vi "2D array sum using for loop.vi"() -> ()   [LabVIEW 2010]
uses:
  <vilib>/Analysis/Matrix/Datatypes/RealMatrix.ctl
  <vilib>/Analysis/Matrix/NI_Matrix.lvlib
panel:
  out "Real Matrix":T1
  in  "Array2":T1
  in  "Array1":T1
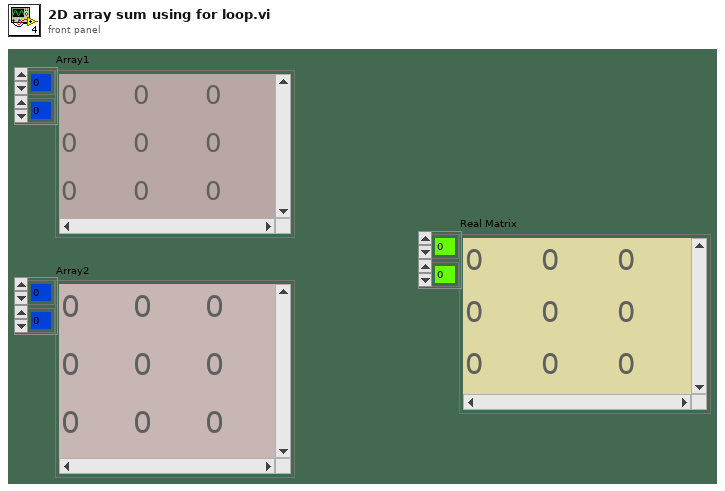
[diagram p1: front panel]
types:
  T1 = typedef "NI_Matrix.lvlib/RealMatrix.ctl" = dbl[][]
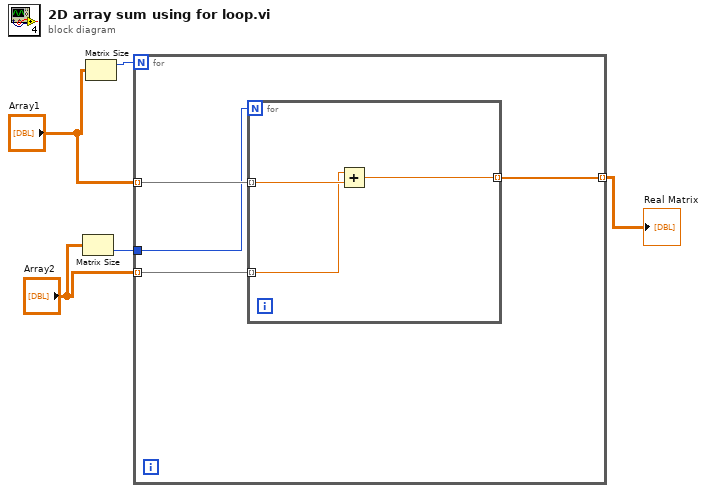
[diagram p0: block diagram]
diagram:
  n1 = Matrix Size(0:"Array2") -> (2:w2:i32)  [unwired: 1 out]
  n2 = Matrix Size(0:"Array1") -> (1:w5:i32)  [unwired: 1 out]
  n3 = for {
    N: w5 -> [_]
    tunnel: "Array1" -> [w9] mode=indexing
    tunnel: [w8] -> w3 mode=indexing
    tunnel: w2 -> [w7]
    tunnel: "Array2" -> [w6] mode=indexing
    n4 = for {
      N: w7 -> [_]
      tunnel: w9 -> [w12] mode=indexing
      tunnel: [w11] -> w8 mode=indexing
      tunnel: w6 -> [w10] mode=indexing
      n5 = Add(x=w10, y=w12) -> (x+y=w11:dbl)
    }
  }
  "Real Matrix" <- w3
